vi "digitalairpressure.vi"() -> ()   [LabVIEW 2021]
uses:
  <vilib>/Instr/_visa.llb/VISA Configure Serial Port (Instr).vi
panel:
  in  "BAÞLAT":bool
  in  "DURDUR":bool
  out "SICAKLIK/ C":dbl(slide) scale=0.0..100.0
  out "GALVANOMETRE":dbl(knob) scale=0.0..100.0
  out "MONOMETRE":dbl(knob) scale=0.0..2000.0
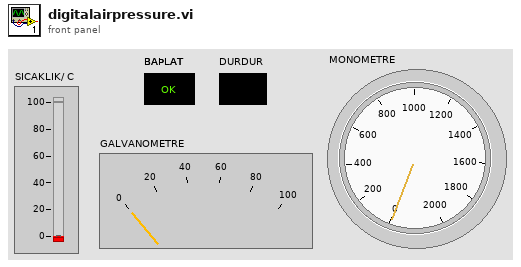
[diagram p1: front panel]
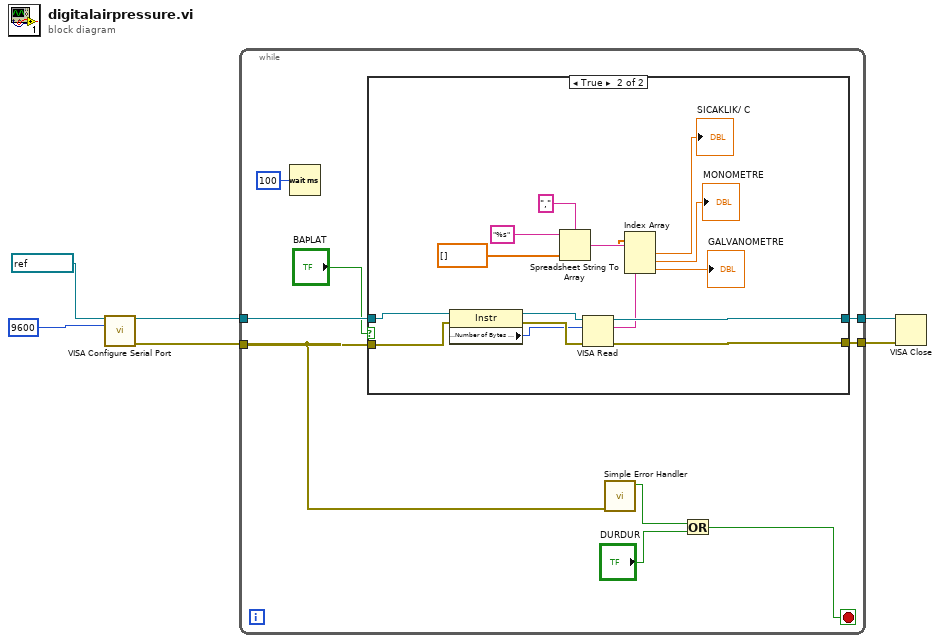
[diagram p0: block diagram]
diagram:
  n1 = call-poly "VISA Configure Serial Port"("VISA resource name"=refnum<visa-resource-name> "COM3", "baud rate (9600)"=u32 9600) -> ("VISA resource name out"=w4:refnum<visa-resource-name>, "error out"=w3:errorcluster)  [unwired: 12 in]
  n2 = while {
    tunnel: w4 -> [w15]
    tunnel: w3 -> [w7]
    tunnel: [w14] -> w6
    tunnel: [w13] -> w5
    stop <- w10 stop-if-true
    n3 = Wait (ms)(milliseconds to wait=u32 100) -> ()  [unwired: 1 out]
    n4 = case shown="True" "BAÞLAT" {
      tunnel: w15 -> [w17 w22]
      tunnel: w7 -> [w16 w21]
      tunnel: [w16 w32] -> w14
      tunnel: [w17 w31] -> w13
      frame False {
      }
      frame True {
        n5 = property class="Instr"(reference=w22, error in=w21) -> (reference out=w19:refnum<visa-resource-name>, error out=w20:errorcluster, "Serial Settings:Number of Bytes at Serial Port"=w18:u32)
        n6 = VISA Read(VISA resource name=w19, byte count=w18, error in (no error)=w20) -> (VISA resource name out=w31:refnum<visa-resource-name>, read buffer=w30:string, error out=w32:errorcluster)  [unwired: 1 out]
        n7 = Spreadsheet String To Array(delimiter (Tab)=",", format string="%s", spreadsheet string=w30, array type (2D Dbl)=dbl[] []) -> (array=w27:dbl[])
        n8 = Index Array(array=w27) -> (element #1=→"SICAKLIK/ C":dbl, element #2=→"MONOMETRE":dbl, element #3=→"GALVANOMETRE":dbl)  [unwired: 3 in]
      }
    }
    n9 = call <vilib>:"Simple Error Handler.vi"("error in (no error)"=w7) -> ("error?"=w12:bool)  [unwired: 4 in, 4 out]
    n10 = Or(x=w12, y="DURDUR") -> (x .or. y?=w10:bool)
  }
  n11 = VISA Close(VISA resource name=w5, error in (no error)=w6) -> ()  [unwired: 1 out]
